vi "PyLoN_SRS5.vi"() -> ()   [LabVIEW 2014]
uses:
  Public/Documents/SIToolkit/LabVIEW/Examples2014_6_0_2_9/Fast Examples/Open-Close Hardware/CamHandle.vi
  <vilib>/Utility/file.llb/Write To Spreadsheet File (I64).vi
  <vilib>/Utility/file.llb/Write To Spreadsheet File (DBL).vi
panel:
  in  "Tab Control":enum32{"Page 1", "Page 2"}(tab)
  in  "Set camera":bool
  in  "stop":bool
  in  "Camera Number":u32=1
  in  "Write Tab Control":T1(tab)
  in  "Frames to collect (nframe)":u32=20000 min=1 step=1
  in  "Apply Timing":bool
  in  "Exposure":dbl min=0.0 step=0.001 format="%.3f"
  in  "Timing Mode":u32(ring)=1 items=["Free Run/Timed"=1, "External Sync/Strobed/Readout per Trigger"=3, "Shift per Trigger (kinetics only)"=13]
  in  "Trigger Edge":u32(ring)=1 items=["Positive Edge"=1, "Negative Edge"=2]
  in  "Collection Mode":u32(ring)=2 items=["Focus"=1, "N-Frame"=2, "Asynchronous"=3]
  in  "ReadOut Mode":u16(ring)=1 items=["Full Frame"=1, "Kinetics"=10]
  in  "Apply Temperature":bool
  in  "Temperature":dbl=-10.0 format="%.2f"
  in  "Apply ADC":bool
  in  "Speed":i32=-2 min=-3 step=1
  in  "Gain":i32(ring)=-1 items=["Don't Change "=-1, "Low"=1, "Medium"=2, "High"=3]
  in  "Offset":i32=-1 min=-1 step=1
  in  "Readout Port":i32(ring)=2 items=["Don't Change"=-1, "Low Noise"=1, "High capacity"=2]
  in  "Apply Shutter":bool
  in  "Open":u32
  in  "Close":u32
  in  "Shutter State":u16(ring)=3 items=["Always Closed"=1, "Open Each Exposure"=2, "Open at Begining of Acquisition"=3, "Open While Waiting for Trigger"=4]
  in  "Apply Cleans":bool
  in  "Final Section Height\n(Minimum Block Size)":u32=100
  in  "Final Section Count\n(Number of Minimum Blocks)":u32=10
  in  "Number of Clean/Clears cycles":u32
  in  "Clean cycle height (Number of \nStrips per Clean/Clear)":u32=100
  in  "Continous Cleans":bool
  in  "Skip Serial Register Clean":bool
  in  "Kinetics Window Height":u32
  in  "Active Y Size":u32=20
  in  "Post Y":u32
  in  "Pre Y":u32
  in  "Active X Size":u32=1340
  in  "Post X":u32
  in  "Pre X":u32
  in  "Vertical Timing Index":u32=1
  in  "Enable / Disable Custom Chip":bool=TRUE
  in  "Apply Custom Chip":bool
  in  "Apply Logic Out":bool
  in  "Logic Output":u16(ring)=1 items=["Not Scan / Not Reading"=1, "Shutter Open"=2, "Not Ready/Busy"=3, "Always Low"=4, "Always High"=8]
  in  "Invert":bool
  in  "Apply ROI":bool
  out "Y Size ROI":u32=20
  out "X Size ROI":u32=1340
  in  "Y Bin":u32=20 min=1 step=1
  in  "Y End":u32=20 min=1 step=1
  in  "Y Start":u32=1 min=1 step=1
  in  "X Bin":u32=1 min=1 step=1
  in  "X End":u32=1340 min=1 max=100000 step=1
  in  "X Start":u32=1 min=1 step=1
  in  "Write Status":string="Ready"
  out "Readout Time":dbl=0.8070999999999999
  in  "Read Camera settings":bool
  out "Temperature 2":dbl=-15.0
  out "Pixel Time\n(1/ADC Speed)":i32=500
  out "Bit Depth":i32=16
  out "ReadOut Port":i32=-1
  out "ADC Offset":i32=-1
  out "ADC Gain":i32=2
  out "ADC Speed":i32=2000
  out "Thermometer":dbl(slide)=-15.0 scale=-100.0..25.0 scale format="%#_6f"
  in  "Read Status":string="Ready"
  out "Camera Ready":bool=TRUE
  out "Vertical Timing":dbl=6.2
  out "Custom Chip Enabled":bool=TRUE
  out "Vertical Index":u32=1
  out "Frame Rate Calc":dbl=1239.003840911907
  in  "Clear Errors":bool
  in  "?":T2(tab)
  in  "?":bool
  in  "Exposure Time (s)":dbl=0.004 min=0.0 step=0.001 format="%.3f"
  in  "?":bool
  in  "?":bool
  out "?":u16[](graph)
  in  "file path":path
  in  "File_name":string
  in  "# of spectrum per frame":i32
  in  "# of Frames":i32
  in  "FLIP SPECTRA":bool
  in  "?":bool
  in  "?":bool
  in  "?":bool
  out "?":dbl[](graph)
  in  "?":bool
  in  "Number of Images":u32=1 min=1 step=1
  out "?":dbl[](graph)
  in  "?":bool
  in  "# of Sets":i32
  out "Current Set":u32=24
  in  "#Ground per set":u32=3
  in  "Timepoints":dbl[](array[numeric])=[200.0, 100.0, 300.0, 400.0, 500.0]
  in  "File Path":path
  in  "File Name":string
  in  "Ground State\nSubstract?":bool
  out "PyLoN Error Out":errorcluster
  out "PyLoN Ready":bool
  out "x/y":dbl
  in  "?":bool
  in  "Write INI Flag":bool
  out "error out":errorcluster
  in  "error in (no error)":errorcluster
  # "Write To Camera"
  # "Read From Camera"
  # "-1 = Item is not supported by this camera"
  # "ms"
  # "°C"
  # "ms"
  # "Timing"
  # "Seconds"
  # "Temperature"
  # "°C"
  # "ADC"
  # "-3 = SLOWEST speed\n-2 = FASTEST speed\n-1 = CURRENT speed (or do not wire)\nOtherwise enter speed in kHz"
  # "Shutter"
  # "Compensation Times"
  # "ms"
  # "Cleans / Clears"
  # "Custom Chip and Timing"
  # "Valid When Kinetics Timing Mode Active"
  # "Logic Output"
  # "Region Of Interest"
  # "REGION OF INTEREST"
  # "TRIGGER"
  # "ADC"
  # "SHUTTER"
  # "INPUT VARIABLES"
  # "TTL LOGIC"
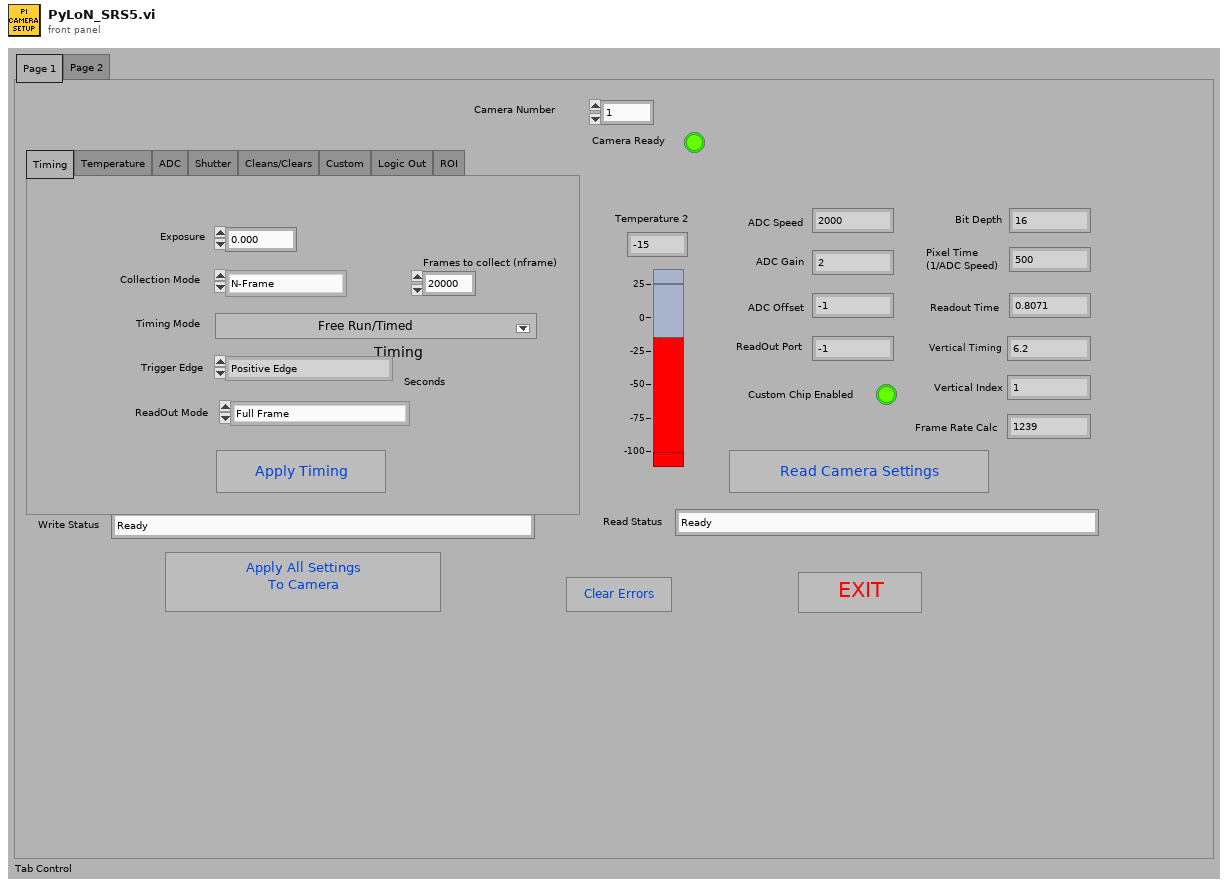
[diagram p1: front panel]
types:
  T1 = enum32{"Timing", "Temperature", "ADC", "Shutter", "Cleans/Clears", "Custom", "Logic Out", "ROI"}
  T2 = enum32{"CONFIGURATION", "RUN", "FOCUS", "FSRS", "SPECTROGRAPH", "ERROR"}
  T3 = cluster{"Pre Y":u32, "Post Y":u32, "Parallel (Y) Size":u32, "Pre X":u32, "Post X":u32, "Serial (X) Size":u32}
  T4 = cluster{"Camera Number":i32, "ROI Number":i32, "X Start":i32, "X End":i32, "X Bin":i32, "Y Start":i32, "Y End":i32, "Y Bin":i32}
  T5 = cluster{"Pre Y":u32, "Post Y":u32, "Active Y":u32, "Pre X":u32, "Post X":u32, "Active X":u32, "Custom Chip Enabled":bool, "Vertical Timing Index":u32}
  T6 = cluster{"Exposure":dbl, "Collection Mode":u32, "Timing Mode":u32, "Trigger Edge":u32, "Temperature":dbl}
  T7 = cluster{"ADC Speed":i32, "ADC Gain":i32, "ADC Offset":i32, "Readout Port":i32, "Num Cleans":u32, "Num Strips per Clean":u32, "Mini Block Size":u32, "Num Min Blocks":u32, "Continous Cleans":bool, "Skip Serial Reg Clean":bool}
  T8 = cluster{"Shutter State":u16, "Open Comp Time ":u32, "Close Comp Time":u32, "Logic Out Setting":u32, "Logic Out Invert":bool}
  T9 = enum32{"Initializing", "RUN", "FSRS", "Monochromator", "Errors"}
  T10 = cluster{"X Start":i32, "X End":i32, "X Bin":i32, "Y Start":i32, "Y End":i32, "Y Bin":i32}
  T11 = cluster{"Value":u32, "Value":u32, "Value":u32, "Value":u32, "Value":u32, "Value":u32}
  T12 = cluster{"acquire focus mode":u32, "Exposure Time (s)":dbl, i32, "Software accumulation":u32}
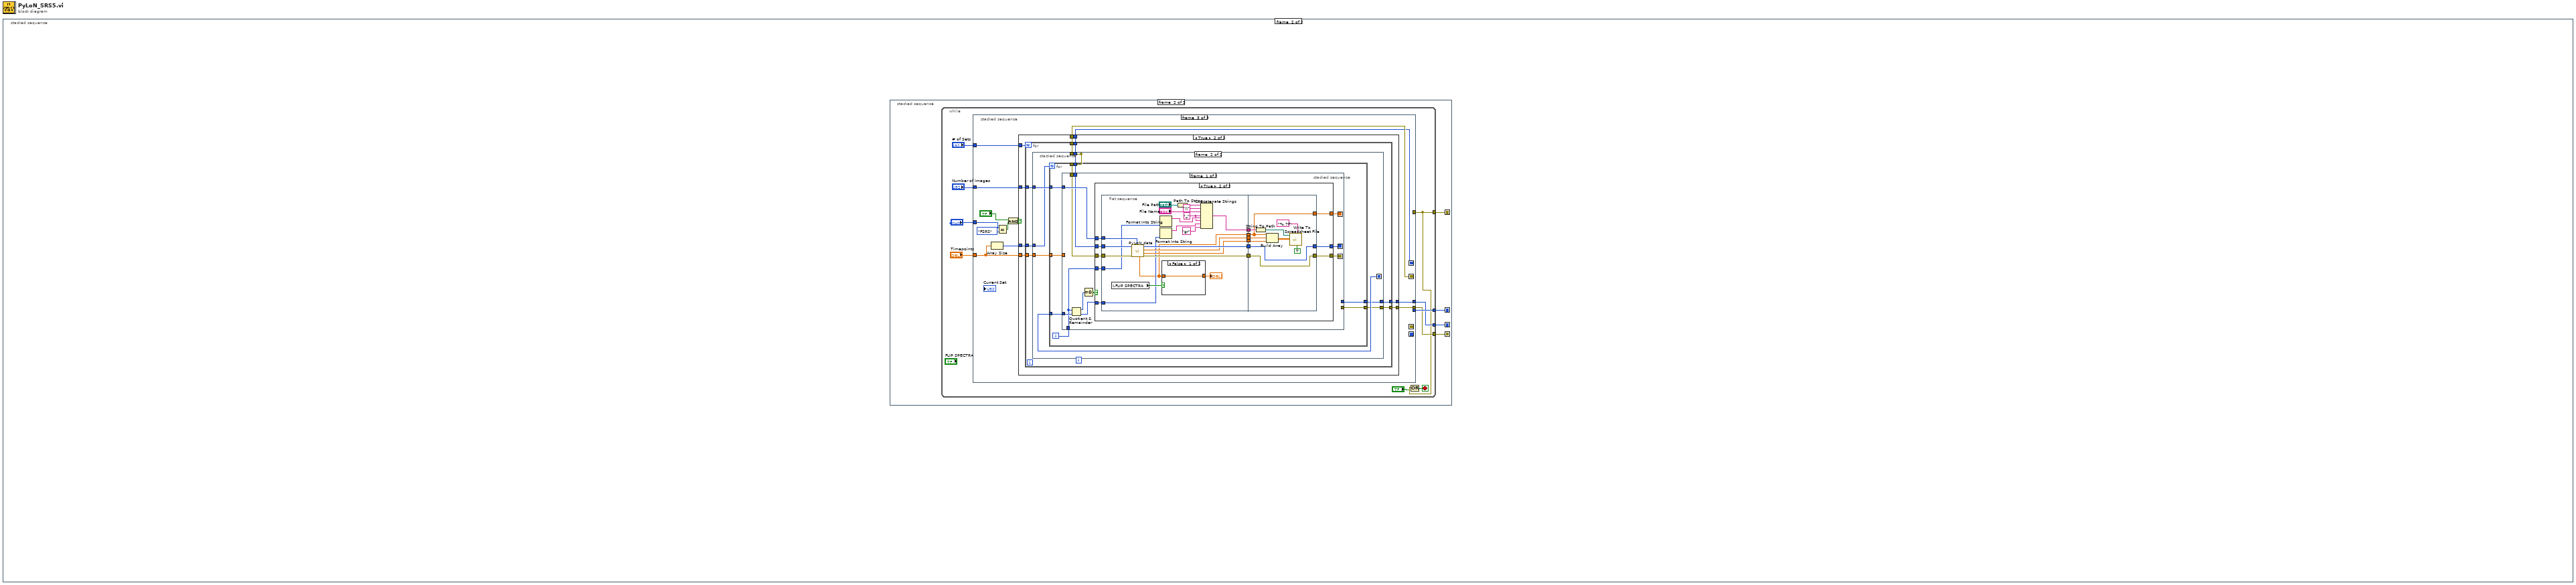
[diagram p0: block diagram]
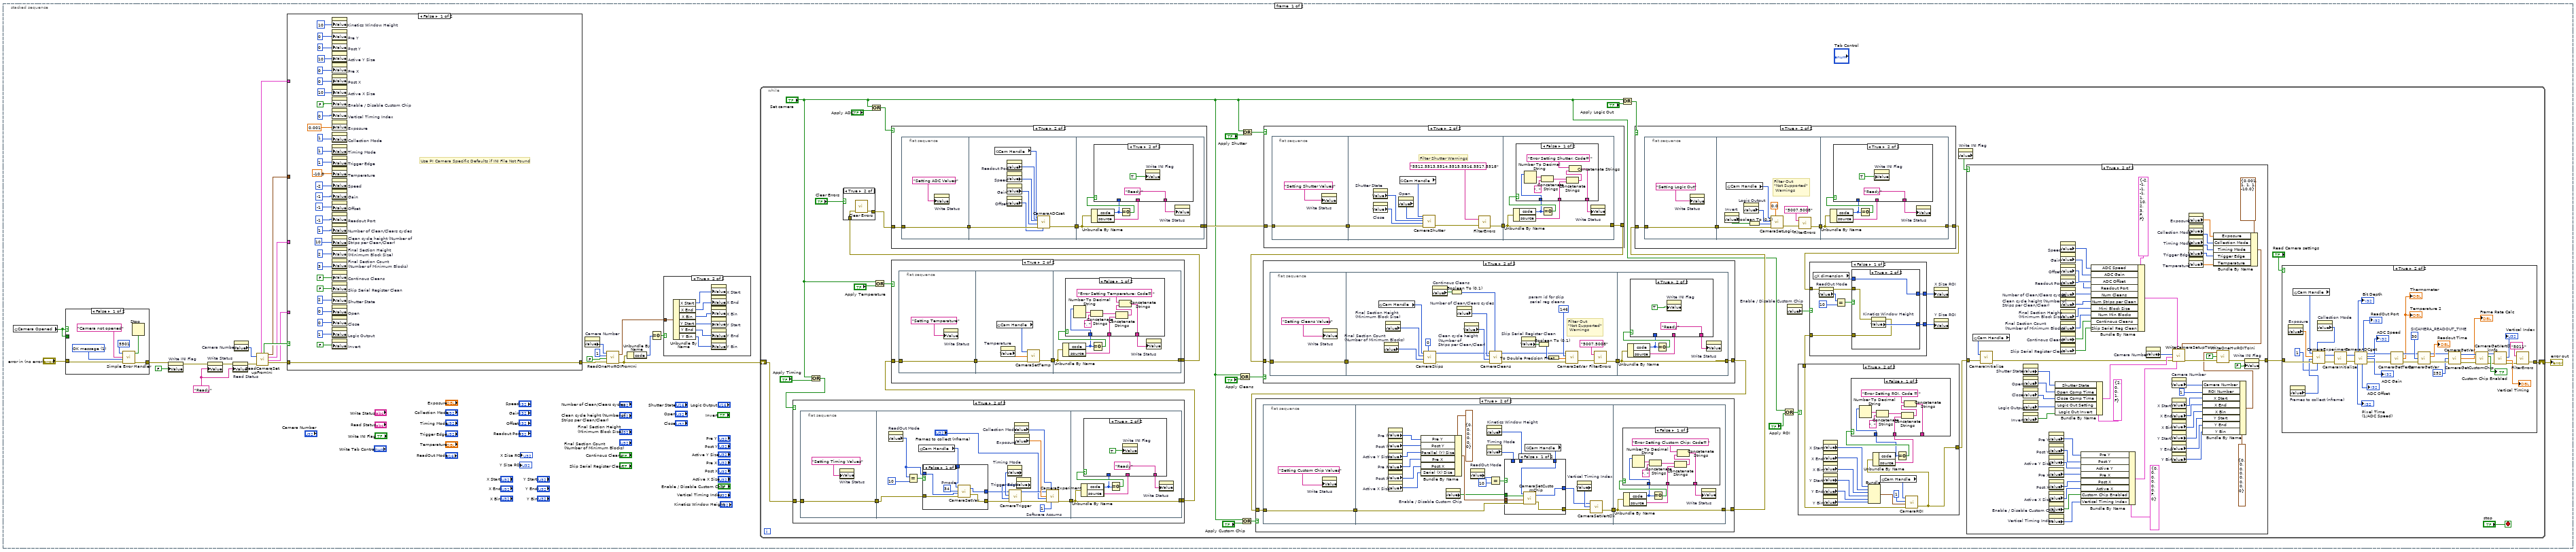
[diagram p2: hidden frame]
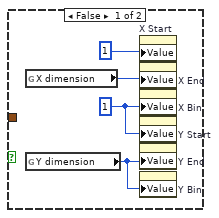
[diagram p3: hidden frame]
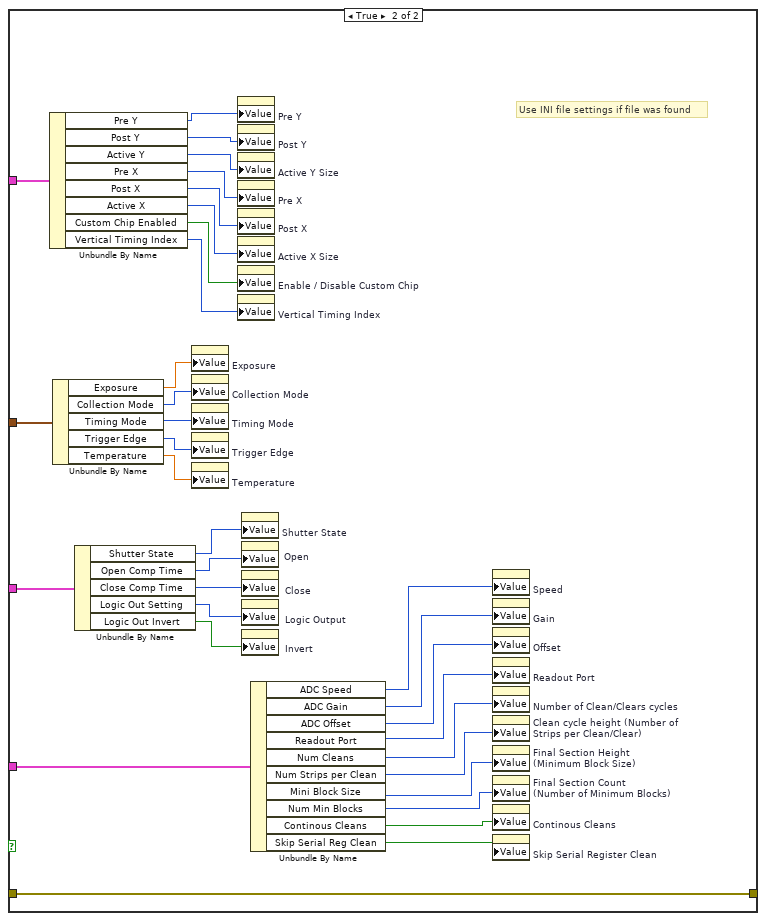
[diagram p4: hidden frame]
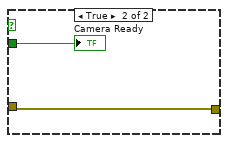
[diagram p5: hidden frame]
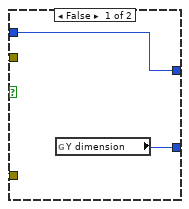
[diagram p7: hidden frame]
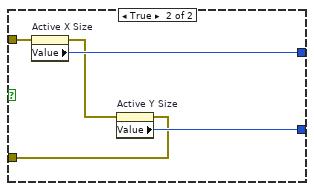
[diagram p8: hidden frame]
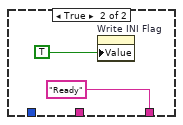
[diagram p10: hidden frame]
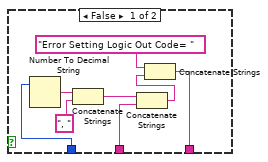
[diagram p12: hidden frame]
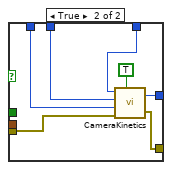
[diagram p14: hidden frame]
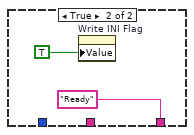
[diagram p15: hidden frame]
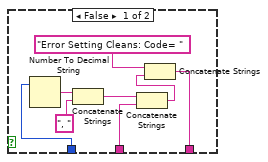
[diagram p17: hidden frame]
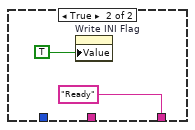
[diagram p19: hidden frame]
diagram:
  n1 = stacked-sequence {
    frame #0 {
      w15 = "Ready"
      n2 = global read "CamHandle.vi" "Camera Opened"() -> (w11:bool)
      n3 = case shown="False" w11 {
        tunnel: [w103 w106] -> w14
        tunnel: "error in (no error)" -> [w99 w106]
        tunnel: w11 -> [_ w105]
        frame False {
          w104 = u16 1 items=["no dialog", "OK message", "continue or stop message"] ("type of dialog (OK msg:1)")
          n4 = call <vilib>:"Simple Error Handler.vi"("error code (no error:0)"=5501, "error source (\" \")"="Camera not opened", "type of dialog (OK msg:1)"=w104, "error in (no error)"=w99) -> ("error?"=w101:bool, "error out"=w103:errorcluster)  [unwired: 1 in, 3 out]
          n5 = Stop(stop? (T)=w101) -> ()
        }
        frame True {
          "Camera Ready" <- w105
        }
      }
      n6 = property on="Write INI Flag" class="Bool (strict)"(error in=w14, "Value"=FALSE) -> (error out=w13:errorcluster)  [unwired: 1 in, 1 out]
      n7 = property on="Write Status" class="Str"(error in=w13, "Value"=w15) -> (error out=w17:errorcluster)  [unwired: 1 in, 1 out]
      n8 = property on="Read Status" class="Str"(error in=w17, "Value"=w15) -> (error out=w16:errorcluster)  [unwired: 1 in, 1 out]
      n9 = property on="Camera Number" class="DigNum (strict)"() -> ("Value"=w8:u32)  [unwired: 2 in, 2 out]
      n10 = call "ReadCameraSetupFromIni.vi"("error in (no error)"=w16, "Camera Number"=w8) -> ("Custom Chip"=w10:T5, "INI File Found"=w22:bool, "error out"=w18:errorcluster, "ADC and Cleans"=w21:T7, "Shutter and Logic Out"=w20:T8, "Timing and Temperature"=w19:T6)
      n11 = case shown="False" w22 {
        tunnel: w19 -> [_ w98]
        tunnel: w20 -> [_ w92]
        tunnel: w21 -> [_ w86]
        tunnel: w18 -> [w45 w75]
        tunnel: [w45 w75] -> w9
        tunnel: w10 -> [_ w74]
        frame False {
          # "Use PI Camera Specific Defaults if INI File Not Found"
          n12 = property on="Kinetics Window Height" class="DigNum (strict)"("Value"=10) -> ()  [unwired: 2 in, 2 out]
          n13 = property on="Pre Y" class="DigNum (strict)"("Value"=0) -> ()  [unwired: 2 in, 2 out]
          n14 = property on="Post Y" class="DigNum (strict)"("Value"=0) -> ()  [unwired: 2 in, 2 out]
          n15 = property on="Active Y Size" class="DigNum (strict)"("Value"=10) -> ()  [unwired: 2 in, 2 out]
          n16 = property on="Pre X" class="DigNum (strict)"("Value"=0) -> ()  [unwired: 2 in, 2 out]
          n17 = property on="Post X" class="DigNum (strict)"("Value"=0) -> ()  [unwired: 2 in, 2 out]
          n18 = property on="Active X Size" class="DigNum (strict)"("Value"=10) -> ()  [unwired: 2 in, 2 out]
          n19 = property on="Enable / Disable Custom Chip" class="Bool (strict)"("Value"=FALSE) -> ()  [unwired: 2 in, 2 out]
          n20 = property on="Vertical Timing Index" class="DigNum (strict)"("Value"=0) -> ()  [unwired: 2 in, 2 out]
          n21 = property on="Exposure" class="DigNum (strict)"("Value"=0.001 ("Exposure")) -> ()  [unwired: 2 in, 2 out]
          n22 = property on="Collection Mode" class="Ring (strict)"("Value"=u32 1 ("Collection Mode")) -> ()  [unwired: 2 in, 2 out]
          n23 = property on="Timing Mode" class="Ring (strict)"("Value"=u32 1 ("Timing Mode")) -> ()  [unwired: 2 in, 2 out]
          n24 = property on="Trigger Edge" class="Ring (strict)"("Value"=u32 1 ("Trigger Edge")) -> ()  [unwired: 2 in, 2 out]
          n25 = property on="Temperature" class="DigNum (strict)"("Value"=-10.0 ("Temperature")) -> ()  [unwired: 2 in, 2 out]
          n26 = property on="Speed" class="DigNum (strict)"("Value"=-2 ("ADC Speed")) -> ()  [unwired: 2 in, 2 out]
          n27 = property on="Gain" class="Ring (strict)"("Value"=-1 ("ADC Gain")) -> ()  [unwired: 2 in, 2 out]
          n28 = property on="Offset" class="DigNum (strict)"("Value"=-1 ("ADC Offset")) -> ()  [unwired: 2 in, 2 out]
          n29 = property on="Readout Port" class="Ring (strict)"("Value"=-1 ("Readout Port")) -> ()  [unwired: 2 in, 2 out]
          n30 = property on="Number of Clean/Clears cycles" class="DigNum (strict)"("Value"=u32 1 ("Num Cleans")) -> ()  [unwired: 2 in, 2 out]
          n31 = property on="Clean cycle height (Number of \nStrips per Clean/Clear)" class="DigNum (strict)"("Value"=u32 10 ("Num Strips per Clean")) -> ()  [unwired: 2 in, 2 out]
          n32 = property on="Final Section Height\n(Minimum Block Size)" class="DigNum (strict)"("Value"=u32 2 ("Mini Block Size")) -> ()  [unwired: 2 in, 2 out]
          n33 = property on="Final Section Count\n(Number of Minimum Blocks)" class="DigNum (strict)"("Value"=u32 3 ("Num Min Blocks")) -> ()  [unwired: 2 in, 2 out]
          n34 = property on="Continous Cleans" class="Bool (strict)"("Value"=FALSE ("Continous Cleans")) -> ()  [unwired: 2 in, 2 out]
          n35 = property on="Skip Serial Register Clean" class="Bool (strict)"("Value"=FALSE ("Skip Serial Reg Clean")) -> ()  [unwired: 2 in, 2 out]
          n36 = property on="Shutter State" class="Ring (strict)"("Value"=u16 2 ("Shutter State")) -> ()  [unwired: 2 in, 2 out]
          n37 = property on="Open" class="DigNum (strict)"("Value"=u32 0 ("Open Comp Time")) -> ()  [unwired: 2 in, 2 out]
          n38 = property on="Close" class="DigNum (strict)"("Value"=u32 0 ("Close Comp Time")) -> ()  [unwired: 2 in, 2 out]
          n39 = property on="Logic Output" class="Ring (strict)"("Value"=u32 1 ("Logic Out Setting")) -> ()  [unwired: 2 in, 2 out]
          n40 = property on="Invert" class="Bool (strict)"("Value"=FALSE ("Logic Out Invert")) -> ()  [unwired: 2 in, 2 out]
        }
        frame True {
          # "Use INI file settings if file was found"
          n41 = Unbundle By Name(w74) -> ("Pre Y"=w73:u32, "Post Y"=w71:u32, "Active Y"=w70:u32, "Pre X"=w69:u32, "Post X"=w72:u32, "Active X"=w68:u32, "Custom Chip Enabled"=w67:bool, "Vertical Timing Index"=w66:u32)
          n42 = Unbundle By Name(w98) -> ("Exposure"=w97:dbl, "Collection Mode"=w96:u32, "Timing Mode"=w95:u32, "Trigger Edge"=w94:u32, "Temperature"=w93:dbl)
          n43 = Unbundle By Name(w92) -> ("Shutter State"=w91:u16, "Open Comp Time"=w90:u32, "Close Comp Time"=w89:u32, "Logic Out Setting"=w88:u32, "Logic Out Invert"=w87:bool)
          n44 = property on="Exposure" class="DigNum (strict)"("Value"=w97) -> ()  [unwired: 2 in, 2 out]
          n45 = property on="Collection Mode" class="Ring (strict)"("Value"=w96) -> ()  [unwired: 2 in, 2 out]
          n46 = property on="Timing Mode" class="Ring (strict)"("Value"=w95) -> ()  [unwired: 2 in, 2 out]
          n47 = property on="Trigger Edge" class="Ring (strict)"("Value"=w94) -> ()  [unwired: 2 in, 2 out]
          n48 = property on="Temperature" class="DigNum (strict)"("Value"=w93) -> ()  [unwired: 2 in, 2 out]
          n49 = property on="Pre Y" class="DigNum (strict)"("Value"=w73) -> ()  [unwired: 2 in, 2 out]
          n50 = property on="Post Y" class="DigNum (strict)"("Value"=w71) -> ()  [unwired: 2 in, 2 out]
          n51 = property on="Active Y Size" class="DigNum (strict)"("Value"=w70) -> ()  [unwired: 2 in, 2 out]
          n52 = property on="Pre X" class="DigNum (strict)"("Value"=w69) -> ()  [unwired: 2 in, 2 out]
          n53 = property on="Post X" class="DigNum (strict)"("Value"=w72) -> ()  [unwired: 2 in, 2 out]
          n54 = property on="Active X Size" class="DigNum (strict)"("Value"=w68) -> ()  [unwired: 2 in, 2 out]
          n55 = property on="Enable / Disable Custom Chip" class="Bool (strict)"("Value"=w67) -> ()  [unwired: 2 in, 2 out]
          n56 = property on="Vertical Timing Index" class="DigNum (strict)"("Value"=w66) -> ()  [unwired: 2 in, 2 out]
          n57 = property on="Shutter State" class="Ring (strict)"("Value"=w91) -> ()  [unwired: 2 in, 2 out]
          n58 = property on="Open" class="DigNum (strict)"("Value"=w90) -> ()  [unwired: 2 in, 2 out]
          n59 = property on="Close" class="DigNum (strict)"("Value"=w89) -> ()  [unwired: 2 in, 2 out]
          n60 = property on="Logic Output" class="Ring (strict)"("Value"=w88) -> ()  [unwired: 2 in, 2 out]
          n61 = property on="Invert" class="Bool (strict)"("Value"=w87) -> ()  [unwired: 2 in, 2 out]
          n62 = Unbundle By Name(w86) -> ("ADC Speed"=w76:i32, "ADC Gain"=w77:i32, "ADC Offset"=w78:i32, "Readout Port"=w79:i32, "Num Cleans"=w80:u32, "Num Strips per Clean"=w81:u32, "Mini Block Size"=w82:u32, "Num Min Blocks"=w83:u32, "Continous Cleans"=w84:bool, "Skip Serial Reg Clean"=w85:bool)
          n63 = property on="Speed" class="DigNum (strict)"("Value"=w76) -> ()  [unwired: 2 in, 2 out]
          n64 = property on="Gain" class="Ring (strict)"("Value"=w77) -> ()  [unwired: 2 in, 2 out]
          n65 = property on="Offset" class="DigNum (strict)"("Value"=w78) -> ()  [unwired: 2 in, 2 out]
          n66 = property on="Readout Port" class="Ring (strict)"("Value"=w79) -> ()  [unwired: 2 in, 2 out]
          n67 = property on="Number of Clean/Clears cycles" class="DigNum (strict)"("Value"=w80) -> ()  [unwired: 2 in, 2 out]
          n68 = property on="Clean cycle height (Number of \nStrips per Clean/Clear)" class="DigNum (strict)"("Value"=w81) -> ()  [unwired: 2 in, 2 out]
          n69 = property on="Final Section Height\n(Minimum Block Size)" class="DigNum (strict)"("Value"=w82) -> ()  [unwired: 2 in, 2 out]
          n70 = property on="Final Section Count\n(Number of Minimum Blocks)" class="DigNum (strict)"("Value"=w83) -> ()  [unwired: 2 in, 2 out]
          n71 = property on="Continous Cleans" class="Bool (strict)"("Value"=w84) -> ()  [unwired: 2 in, 2 out]
          n72 = property on="Skip Serial Register Clean" class="Bool (strict)"("Value"=w85) -> ()  [unwired: 2 in, 2 out]
        }
      }
      n73 = property on="Camera Number" class="DigNum (strict)"() -> ("Value"=w7:u32)  [unwired: 2 in, 2 out]
      n74 = call "ReadOneHwROIFromIni.vi"("error in (no error)"=w9, "Show Message"=FALSE, "ROI Number"=1, "Camera Number"=w7) -> ("error out"=w4:errorcluster, "ROI Values"=w1:T10)
      n75 = Unbundle By Name(w4) -> ("code"=w2:i32)
      n76 = Equal To 0?(x=w2) -> (x = 0?=w3:bool)
      n77 = case shown="True" w3 {
        tunnel: w1 -> [_ w35]
        frame False {
          w26 = 1
          n78 = global read "CamHandle.vi" "X dimension"() -> (w27:u32)
          n79 = global read "CamHandle.vi" "Y dimension"() -> (w25:u32)
          n80 = property on="X Start" class="DigNum (strict)"("Value"=1) -> ()  [unwired: 2 in, 2 out]
          n81 = property on="X End" class="DigNum (strict)"("Value"=w27) -> ()  [unwired: 2 in, 2 out]
          n82 = property on="X Bin" class="DigNum (strict)"("Value"=w26) -> ()  [unwired: 2 in, 2 out]
          n83 = property on="Y Start" class="DigNum (strict)"("Value"=w26) -> ()  [unwired: 2 in, 2 out]
          n84 = property on="Y End" class="DigNum (strict)"("Value"=w25) -> ()  [unwired: 2 in, 2 out]
          n85 = property on="Y Bin" class="DigNum (strict)"("Value"=w25) -> ()  [unwired: 2 in, 2 out]
        }
        frame True {
          n86 = Unbundle By Name(w35) -> ("X Start"=w34:i32, "X End"=w33:i32, "X Bin"=w32:i32, "Y Start"=w31:i32, "Y End"=w30:i32, "Y Bin"=w29:i32)
          n87 = property on="X Start" class="DigNum (strict)"("Value"=w34) -> ()  [unwired: 2 in, 2 out]
          n88 = property on="X End" class="DigNum (strict)"("Value"=w33) -> ()  [unwired: 2 in, 2 out]
          n89 = property on="X Bin" class="DigNum (strict)"("Value"=w32) -> ()  [unwired: 2 in, 2 out]
          n90 = property on="Y Start" class="DigNum (strict)"("Value"=w31) -> ()  [unwired: 2 in, 2 out]
          n91 = property on="Y End" class="DigNum (strict)"("Value"=w30) -> ()  [unwired: 2 in, 2 out]
          n92 = property on="Y Bin" class="DigNum (strict)"("Value"=w29) -> ()  [unwired: 2 in, 2 out]
        }
      }
      n93 = while {
        shift-right: [w141] -> w23
        shift-left: w4 -> [w137]
        stop <- "stop" stop-if-true
        n94 = Or(x="Set camera", y="Apply Timing") -> (x .or. y?=w138:bool)
        n95 = case shown="True" w138 {
          tunnel: w137 -> [w463 w467]
          tunnel: [w463 w464] -> w135
          frame False {
          }
          frame True {
            n96 = flat-sequence {
              tunnel: w467 -> [w469]
              tunnel: [w469] -> w466
              tunnel: w466 -> [w474]
              tunnel: [w478] -> w465
              tunnel: w465 -> [w498]
              tunnel: [w498] -> w464
              frame #0 {
                n97 = property on="Write Status" class="Str"("Value"="Setting Timing Values") -> ()  [unwired: 2 in, 2 out]
              }
              frame #1 {
                w483 = 1  # Software Accums
                n98 = property on="ReadOut Mode" class="Ring (strict)"() -> ("Value"=w471:u16)  [unwired: 2 in, 2 out]
                n99 = Equal?(x=w471, y=10) -> (x = y?=w473:bool)
                n100 = global read "CamHandle.vi" "Cam Handle"() -> (w475:u32)
                n101 = case shown="False" w473 {
                  tunnel: [w490 w492] -> w477
                  tunnel: [w489 w493] -> w476
                  tunnel: w475 -> [w488 w493]
                  tunnel: w474 -> [w487 w492]
                  tunnel: w471 -> [w486 _]
                  frame False {
                    w491 = 34  # Pmode
                    n102 = call <userlib>:"CameraSetVar.vi"("error in"=w487, "Value"=w486, "Parameter ID"=w491, "Camera Handle"=w488) -> ("error out"=w490:errorcluster, "CameraHandle"=w489:u32)
                  }
                  frame True {
                  }
                }
                n103 = property on="Timing Mode" class="Ring (strict)"() -> ("Value"=w485:u32)  [unwired: 2 in, 2 out]
                n104 = property on="Collection Mode" class="Ring (strict)"() -> ("Value"=w482:u32)  [unwired: 2 in, 2 out]
                n105 = property on="Exposure" class="DigNum (strict)"() -> ("Value"=w484:dbl)  [unwired: 2 in, 2 out]
                n106 = property on="Trigger Edge" class="Ring (strict)"() -> ("Value"=w480:u32)  [unwired: 2 in, 2 out]
                n107 = call <userlib>:"CameraTrigger.vi"("error in"=w477, "Trigger Edge"=w480, "Timing Mode"=w485, "Camera Handle"=w476) -> ("error out"=w479:errorcluster, "Camera Handle"=w481:u32)
                n108 = call <userlib>:"CameraExperiment.vi"("Number of Accumulations"=w483, "Acquire / Focus Flag"=w482, "error in"=w479, "Number of Images"="Frames to collect (nframe)", "Exposure (sec)"=w484, "Camera Handle"=w481) -> ("error out"=w478:errorcluster)  [unwired: 1 out]
              }
              frame #2 {
                n109 = Unbundle By Name(w498) -> ("code"=w494:i32, "source"=w495:string)
                n110 = Equal To 0?(x=w494) -> (x = 0?=w497:bool)
                n111 = case shown="True" w497 {
                  tunnel: [w499 "Ready"] -> w496
                  tunnel: w495 -> [w500 _]
                  tunnel: w494 -> [w505 _]
                  frame False {
                    n112 = Number To Decimal String(number=w505) -> (decimal integer string=w504:string)  [unwired: 1 in]
                    n113 = Concatenate Strings(w504, ", ") -> (w501:string)
                    n114 = Concatenate Strings(w501, w500) -> (w502:string)
                    n115 = Concatenate Strings("Error Setting Timing: Code= ", w502) -> (w499:string)
                  }
                  frame True {
                    n116 = property on="Write INI Flag" class="Bool (strict)"("Value"=TRUE) -> ()  [unwired: 2 in, 2 out]
                  }
                }
                n117 = property on="Write Status" class="Str"("Value"=w496) -> ()  [unwired: 2 in, 2 out]
              }
            }
          }
        }
        n118 = Or(x="Set camera", y="Apply ADC") -> (x .or. y?=w133:bool)
        n119 = Or(x="Set camera", y="Apply Temperature") -> (x .or. y?=w136:bool)
        n120 = case shown="True" w136 {
          tunnel: w135 -> [w437 w441]
          tunnel: [w437 w438] -> w111
          frame False {
          }
          frame True {
            n121 = flat-sequence {
              tunnel: w441 -> [w443]
              tunnel: [w443] -> w440
              tunnel: w440 -> [w445]
              tunnel: [w444] -> w439
              tunnel: w439 -> [w452]
              tunnel: [w452] -> w438
              frame #0 {
                n122 = property on="Write Status" class="Str"("Value"="Setting Temperature") -> ()  [unwired: 2 in, 2 out]
              }
              frame #1 {
                n123 = global read "CamHandle.vi" "Cam Handle"() -> (w446:u32)
                n124 = property on="Temperature" class="DigNum (strict)"() -> ("Value"=w447:dbl)  [unwired: 2 in, 2 out]
                n125 = call <userlib>:"CameraSetTemp.vi"("error in (no error)"=w445, "Temperature"=w447, "Camera Handle"=w446) -> ("error out"=w444:errorcluster)  [unwired: 1 out]
              }
              frame #2 {
                n126 = Unbundle By Name(w452) -> ("code"=w449:i32, "source"=w450:string)
                n127 = Equal To 0?(x=w449) -> (x = 0?=w451:bool)
                n128 = case shown="False" w451 {
                  tunnel: [w453 "Ready"] -> w448
                  tunnel: w450 -> [w454 _]
                  tunnel: w449 -> [w459 _]
                  frame False {
                    n129 = Number To Decimal String(number=w459) -> (decimal integer string=w458:string)  [unwired: 1 in]
                    n130 = Concatenate Strings(w458, ", ") -> (w455:string)
                    n131 = Concatenate Strings(w455, w454) -> (w456:string)
                    n132 = Concatenate Strings("Error Setting Temperature: Code= ", w456) -> (w453:string)
                  }
                  frame True {
                    n133 = property on="Write INI Flag" class="Bool (strict)"("Value"=TRUE) -> ()  [unwired: 2 in, 2 out]
                  }
                }
                n134 = property on="Write Status" class="Str"("Value"=w448) -> ()  [unwired: 2 in, 2 out]
              }
            }
          }
        }
        n135 = case shown="True" "Clear Errors" {
          tunnel: w111 -> [w144 w146]
          tunnel: [w144 w145] -> w110
          frame False {
          }
          frame True {
            n136 = call <vilib>:"Clear Errors.vi"("error in (no error)"=w146) -> ("error out"=w145:errorcluster)  [unwired: 5 in, 1 out]
          }
        }
        n137 = case shown="True" w133 {
          tunnel: w110 -> [w351 w355]
          tunnel: [w351 w352] -> w132
          frame False {
          }
          frame True {
            n138 = flat-sequence {
              tunnel: w355 -> [w357]
              tunnel: [w357] -> w354
              tunnel: w354 -> [w361]
              tunnel: [w360] -> w353
              tunnel: w353 -> [w366]
              tunnel: [w366] -> w352
              frame #0 {
                n139 = property on="Write Status" class="Str"("Value"="Setting ADC Values") -> ()  [unwired: 2 in, 2 out]
              }
              frame #1 {
                n140 = global read "CamHandle.vi" "Cam Handle"() -> (w358:u32)
                n141 = property on="Readout Port" class="Ring (strict)"() -> ("Value"=w362:i32)  [unwired: 2 in, 2 out]
                n142 = property on="Speed" class="DigNum (strict)"() -> ("Value"=w363:i32)  [unwired: 2 in, 2 out]
                n143 = property on="Gain" class="Ring (strict)"() -> ("Value"=w364:i32)  [unwired: 2 in, 2 out]
                n144 = property on="Offset" class="DigNum (strict)"() -> ("Value"=w359:i32)  [unwired: 2 in, 2 out]
                n145 = call <userlib>:"CameraADCset.vi"("ADC offset"=w359, "Read Out port"=w362, "error in (no error)"=w361, "ADC Gain"=w364, "ADC Speed"=w363, "Camera Handle"=w358) -> ("error out"=w360:errorcluster)  [unwired: 1 out]
              }
              frame #2 {
                n146 = Unbundle By Name(w366) -> ("code"=w367:i32, "source"=w368:string)
                n147 = Equal To 0?(x=w367) -> (x = 0?=w369:bool)
                n148 = case shown="True" w369 {
                  tunnel: [w370 "Ready"] -> w365
                  tunnel: w368 -> [w371 _]
                  tunnel: w367 -> [w376 _]
                  frame False {
                    n149 = Number To Decimal String(number=w376) -> (decimal integer string=w375:string)  [unwired: 1 in]
                    n150 = Concatenate Strings(w375, ", ") -> (w372:string)
                    n151 = Concatenate Strings(w372, w371) -> (w373:string)
                    n152 = Concatenate Strings("Error Setting ADC: Code= ", w373) -> (w370:string)
                  }
                  frame True {
                    n153 = property on="Write INI Flag" class="Bool (strict)"("Value"=TRUE) -> ()  [unwired: 2 in, 2 out]
                  }
                }
                n154 = property on="Write Status" class="Str"("Value"=w365) -> ()  [unwired: 2 in, 2 out]
              }
            }
          }
        }
        n155 = Or(x="Set camera", y="Apply Cleans") -> (x .or. y?=w127:bool)
        n156 = Or(x="Set camera", y="Apply Custom Chip") -> (x .or. y?=w124:bool)
        n157 = Or(x="Set camera", y="Apply Shutter") -> (x .or. y?=w129:bool)
        n158 = case shown="True" w129 {
          tunnel: w132 -> [w321 w325]
          tunnel: [w321 w322] -> w128
          frame False {
          }
          frame True {
            n159 = flat-sequence {
              tunnel: w325 -> [w327]
              tunnel: [w327] -> w324
              tunnel: w324 -> [w331]
              tunnel: [w329] -> w323
              tunnel: w323 -> [w340]
              tunnel: [w340] -> w322
              frame #0 {
                n160 = property on="Write Status" class="Str"("Value"="Setting Shutter Values") -> ()  [unwired: 2 in, 2 out]
              }
              frame #1 {
                # "Filter Shutter Warnings"
                n161 = property on="Shutter State" class="Ring (strict)"() -> ("Value"=w334:u16)  [unwired: 2 in, 2 out]
                n162 = property on="Close" class="DigNum (strict)"() -> ("Value"=w332:u32)  [unwired: 2 in, 2 out]
                n163 = property on="Open" class="DigNum (strict)"() -> ("Value"=w333:u32)  [unwired: 2 in, 2 out]
                n164 = global read "CamHandle.vi" "Cam Handle"() -> (w328:u32)
                n165 = call <userlib>:"CameraShutter.vi"("Camera Handle"=w328, "Shutter Comp Time: Pre Open"=w333, "Shutter Comp Time: Post Open"=w332, "error in"=w331, "Shutter State"=w334) -> ("error out"=w330:errorcluster)  [unwired: 1 out]
                n166 = call "FilterErrors.vi"("error in (no error)"=w330, "Error Numbers To Filter"="5512,5513,5514,5515,5516,5517,5518") -> ("error out"=w329:errorcluster)
              }
              frame #2 {
                n167 = Unbundle By Name(w340) -> ("code"=w337:i32, "source"=w338:string)
                n168 = Equal To 0?(x=w337) -> (x = 0?=w339:bool)
                n169 = case shown="False" w339 {
                  tunnel: [w341 "Ready"] -> w336
                  tunnel: w338 -> [w342 _]
                  tunnel: w337 -> [w347 _]
                  frame False {
                    n170 = Number To Decimal String(number=w347) -> (decimal integer string=w346:string)  [unwired: 1 in]
                    n171 = Concatenate Strings(w346, ", ") -> (w343:string)
                    n172 = Concatenate Strings(w343, w342) -> (w344:string)
                    n173 = Concatenate Strings("Error Setting Shutter: Code= ", w344) -> (w341:string)
                  }
                  frame True {
                    n174 = property on="Write INI Flag" class="Bool (strict)"("Value"=TRUE) -> ()  [unwired: 2 in, 2 out]
                  }
                }
                n175 = property on="Write Status" class="Str"("Value"=w336) -> ()  [unwired: 2 in, 2 out]
              }
            }
          }
        }
        n176 = case shown="True" w127 {
          tunnel: w128 -> [w279 w283]
          tunnel: [w279 w280] -> w125
          frame False {
          }
          frame True {
            n177 = flat-sequence {
              tunnel: w283 -> [w285]
              tunnel: [w285] -> w282
              tunnel: w282 -> [w298]
              tunnel: [w286] -> w281
              tunnel: w281 -> [w310]
              tunnel: [w310] -> w280
              frame #0 {
                n178 = property on="Write Status" class="Str"("Value"="Setting Cleans Values") -> ()  [unwired: 2 in, 2 out]
              }
              frame #1 {
                w290 = u32 146  # param id for skip  serial reg cleans
                # "Filter Out\n\"Not Supported\"\n Warnings"
                n179 = global read "CamHandle.vi" "Cam Handle"() -> (w299:u32)
                n180 = property on="Final Section Count\n(Number of Minimum Blocks)" class="DigNum (strict)"() -> ("Value"=w304:u32)  [unwired: 2 in, 2 out]
                n181 = property on="Final Section Height\n(Minimum Block Size)" class="DigNum (strict)"() -> ("Value"=w305:u32)  [unwired: 2 in, 2 out]
                n182 = call <userlib>:"CameraSkips.vi"("Camera Handle"=w299, "Minimum Block Size"=w305, "Number of Minimum blocks"=w304, "error in"=w298, "Type of Skips"=u32 0) -> ("Camera Handle"=w295:u32, "error out"=w296:errorcluster)
                n183 = property on="Continous Cleans" class="Bool (strict)"() -> ("Value"=w302:bool)  [unwired: 2 in, 2 out]
                n184 = Boolean To (0,1)(Boolean=w302) -> (0, 1=w297:i16)
                n185 = property on="Number of Clean/Clears cycles" class="DigNum (strict)"() -> ("Value"=w301:u32)  [unwired: 2 in, 2 out]
                n186 = property on="Clean cycle height (Number of \nStrips per Clean/Clear)" class="DigNum (strict)"() -> ("Value"=w300:u32)  [unwired: 2 in, 2 out]
                n187 = call <userlib>:"CameraCleans.vi"("Camera Handle"=w295, "Number of Clears"=w301, "Number of Strips Per Clear"=w300, "error in"=w296, "Continuous Clears"=w297) -> ("Camera Handle"=w287:u32, "error out"=w288:errorcluster)
                n188 = property on="Skip Serial Register Clean" class="Bool (strict)"() -> ("Value"=w292:bool)  [unwired: 2 in, 2 out]
                n189 = Boolean To (0,1)(Boolean=w292) -> (0, 1=w291:i16)
                n190 = To Double Precision Float(number=w291) -> (double precision float=w293:dbl)
                n191 = call <userlib>:"CameraSetVar.vi"("error in"=w288, "Value"=w293, "Parameter ID"=w290, "Camera Handle"=w287) -> ("error out"=w289:errorcluster)  [unwired: 1 out]
                n192 = call "FilterErrors.vi"("error in (no error)"=w289, "Error Numbers To Filter"="5007,5008") -> ("error out"=w286:errorcluster)
              }
              frame #2 {
                n193 = Unbundle By Name(w310) -> ("code"=w307:i32, "source"=w308:string)
                n194 = Equal To 0?(x=w307) -> (x = 0?=w309:bool)
                n195 = case shown="True" w309 {
                  tunnel: [w311 "Ready"] -> w306
                  tunnel: w308 -> [w312 _]
                  tunnel: w307 -> [w317 _]
                  frame False {
                    n196 = Number To Decimal String(number=w317) -> (decimal integer string=w316:string)  [unwired: 1 in]
                    n197 = Concatenate Strings(w316, ", ") -> (w313:string)
                    n198 = Concatenate Strings(w313, w312) -> (w314:string)
                    n199 = Concatenate Strings("Error Setting Cleans: Code= ", w314) -> (w311:string)
                  }
                  frame True {
                    n200 = property on="Write INI Flag" class="Bool (strict)"("Value"=TRUE) -> ()  [unwired: 2 in, 2 out]
                  }
                }
                n201 = property on="Write Status" class="Str"("Value"=w306) -> ()  [unwired: 2 in, 2 out]
              }
            }
          }
        }
        n202 = case shown="True" w124 {
          tunnel: w125 -> [w224 w228]
          tunnel: [w224 w225] -> w122
          frame False {
          }
          frame True {
            n203 = flat-sequence {
              tunnel: w228 -> [w230]
              tunnel: [w230] -> w227
              tunnel: w227 -> [w245]
              tunnel: [w250] -> w226
              tunnel: w226 -> [w268]
              tunnel: [w268] -> w225
              frame #0 {
                n204 = property on="Write Status" class="Str"("Value"="Setting Custom Chip Values") -> ()  [unwired: 2 in, 2 out]
              }
              frame #1 {
                n205 = property on="Pre Y" class="DigNum (strict)"() -> ("Value"=w236:u32)  [unwired: 2 in, 2 out]
                n206 = property on="Post Y" class="DigNum (strict)"() -> ("Value"=w235:u32)  [unwired: 2 in, 2 out]
                n207 = property on="Active Y Size" class="DigNum (strict)"() -> ("Value"=w234:u32)  [unwired: 2 in, 2 out]
                n208 = property on="Pre X" class="DigNum (strict)"() -> ("Value"=w232:u32)  [unwired: 2 in, 2 out]
                n209 = property on="Post X" class="DigNum (strict)"() -> ("Value"=w231:u32)  [unwired: 2 in, 2 out]
                n210 = property on="Active X Size" class="DigNum (strict)"() -> ("Value"=w233:u32)  [unwired: 2 in, 2 out]
                n211 = Bundle By Name(cluster=T3 {"Pre Y"=0, "Post Y"=0, "Parallel (Y) Size"=0, "Pre X"=0, "Post X"=0, "Serial (X) Size"=0} ("Custom Chip Settings"), "Pre Y"=w236, "Post Y"=w235, "Parallel (Y) Size"=w234, "Pre X"=w232, "Post X"=w231, "Serial (X) Size"=w233) -> (w239:T3)
                n212 = property on="Enable / Disable Custom Chip" class="Bool (strict)"() -> ("Value"=w238:bool)  [unwired: 2 in, 2 out]
                n213 = property on="ReadOut Mode" class="Ring (strict)"() -> ("Value"=w248:u16)  [unwired: 2 in, 2 out]
                n214 = property on="Kinetics Window Height" class="DigNum (strict)"() -> ("Value"=w244:u32)  [unwired: 2 in, 2 out]
                n215 = property on="Timing Mode" class="Ring (strict)"() -> ("Value"=w243:u32)  [unwired: 2 in, 2 out]
                n216 = Equal?(x=w248, y=10) -> (x = y?=w247:bool)
                n217 = global read "CamHandle.vi" "Cam Handle"() -> (w242:u32)
                n218 = case shown="False" w247 {
                  tunnel: w245 -> [w256 w263]
                  tunnel: [w255 w262] -> w241
                  tunnel: w244 -> [_ w260]
                  tunnel: w243 -> [_ w259]
                  tunnel: w242 -> [w254 w258]
                  tunnel: w239 -> [w253 _]
                  tunnel: w238 -> [w252 _]
                  tunnel: [w251 w257] -> w237
                  frame False {
                    n219 = call <userlib>:"CameraSetCustomChip.vi"("error in (no error)"=w256, "Custom Chip Settings"=w253, "Enable/Disable Custom Chip"=w252, "Camera Handle"=w254) -> ("error out"=w255:errorcluster, "Camera Handle"=w251:u32)
                  }
                  frame True {
                    n220 = call <userlib>:"CameraKinetics.vi"("Camera Handle"=w258, "Window Size"=w260, "TriggerMode"=w259, "error in (no error)"=w263, "Enable/Disable Kinetics"=TRUE) -> ("Camera Handle"=w257:u32, "error out"=w262:errorcluster)
                  }
                }
                n221 = property on="Vertical Timing Index" class="DigNum (strict)"() -> ("Value"=w249:u32)  [unwired: 2 in, 2 out]
                n222 = call <userlib>:"CameraSetVertClk.vi"("error in (no error)"=w241, "Vertical Clock"=w249, "Camera Handle"=w237) -> ("error out"=w250:errorcluster)  [unwired: 1 out]
              }
              frame #2 {
                n223 = Unbundle By Name(w268) -> ("code"=w265:i32, "source"=w266:string)
                n224 = Equal To 0?(x=w265) -> (x = 0?=w267:bool)
                n225 = case shown="False" w267 {
                  tunnel: [w269 "Ready"] -> w264
                  tunnel: w266 -> [w270 _]
                  tunnel: w265 -> [w275 _]
                  frame False {
                    n226 = Number To Decimal String(number=w275) -> (decimal integer string=w274:string)  [unwired: 1 in]
                    n227 = Concatenate Strings(w274, ", ") -> (w271:string)
                    n228 = Concatenate Strings(w271, w270) -> (w272:string)
                    n229 = Concatenate Strings("Error Setting Clustom Chip: Code= ", w272) -> (w269:string)
                  }
                  frame True {
                    n230 = property on="Write INI Flag" class="Bool (strict)"("Value"=TRUE) -> ()  [unwired: 2 in, 2 out]
                  }
                }
                n231 = property on="Write Status" class="Str"("Value"=w264) -> ()  [unwired: 2 in, 2 out]
              }
            }
          }
        }
        n232 = Or(x="Set camera", y="Apply Logic Out") -> (x .or. y?=w121:bool)
        n233 = case shown="True" w121 {
          tunnel: w122 -> [w193 w197]
          tunnel: [w193 w194] -> w115
          frame False {
          }
          frame True {
            n234 = flat-sequence {
              tunnel: w197 -> [w199]
              tunnel: [w199] -> w196
              tunnel: w196 -> [w204]
              tunnel: [w200] -> w195
              tunnel: w195 -> [w213]
              tunnel: [w213] -> w194
              frame #0 {
                n235 = property on="Write Status" class="Str"("Value"="Setting Logic Out") -> ()  [unwired: 2 in, 2 out]
              }
              frame #1 {
                # "Filter Out\n\"Not Supported\"\n Warnings"
                n236 = property on="Invert" class="Bool (strict)"() -> ("Value"=w206:bool)  [unwired: 2 in, 2 out]
                n237 = global read "CamHandle.vi" "Cam Handle"() -> (w203:u32)
                n238 = property on="Logic Output" class="Ring (strict)"() -> ("Value"=w208:u16)  [unwired: 2 in, 2 out]
                n239 = Boolean To (0,1)(Boolean=w206) -> (0, 1=w207:i16)
                n240 = call <userlib>:"CameraSetLogic.vi"("Reserved"=0.0, "error in (no error)"=w204, "Invert Logic"=w207, "Logic Output"=w208, "Camera Handle"=w203) -> ("error out"=w201:errorcluster)  [unwired: 1 in, 1 out]
                n241 = call "FilterErrors.vi"("error in (no error)"=w201, "Error Numbers To Filter"="5007,5008") -> ("error out"=w200:errorcluster)
              }
              frame #2 {
                n242 = Unbundle By Name(w213) -> ("code"=w210:i32, "source"=w211:string)
                n243 = Equal To 0?(x=w210) -> (x = 0?=w212:bool)
                n244 = case shown="True" w212 {
                  tunnel: [w214 "Ready"] -> w209
                  tunnel: w211 -> [w215 _]
                  tunnel: w210 -> [w220 _]
                  frame False {
                    n245 = Number To Decimal String(number=w220) -> (decimal integer string=w219:string)  [unwired: 1 in]
                    n246 = Concatenate Strings(w219, ", ") -> (w216:string)
                    n247 = Concatenate Strings(w216, w215) -> (w217:string)
                    n248 = Concatenate Strings("Error Setting Logic Out Code= ", w217) -> (w214:string)
                  }
                  frame True {
                    n249 = property on="Write INI Flag" class="Bool (strict)"("Value"=TRUE) -> ()  [unwired: 2 in, 2 out]
                  }
                }
                n250 = property on="Write Status" class="Str"("Value"=w209) -> ()  [unwired: 2 in, 2 out]
              }
            }
          }
        }
        n251 = Or(x="Set camera", y="Apply ROI") -> (x .or. y?=w109:bool)
        n252 = property on="Enable / Disable Custom Chip" class="Bool (strict)"() -> ("Value"=w118:bool)  [unwired: 2 in, 2 out]
        n253 = case shown="False" w118 {
          tunnel: [w151 w167] -> w117
          tunnel: [w150 w166] -> w116
          tunnel: w115 -> [w149 w165]
          tunnel: [w147 w163] -> w114
          frame False {
            n254 = global read "CamHandle.vi" "X dimension"() -> (w152:u32)
            n255 = property on="ReadOut Mode" class="Ring (strict)"(error in=w149) -> (error out=w148:errorcluster, "Value"=w153:u16)  [unwired: 1 in, 1 out]
            n256 = Equal?(x=w153, y=10) -> (x = y?=w154:bool)
            n257 = case shown="True" w154 {
              tunnel: w152 -> [w158 w162]
              tunnel: [w158 w162] -> w151
              tunnel: [w157 w161] -> w150
              tunnel: w148 -> [w156 w160]
              tunnel: [w156 w159] -> w147
              frame False {
                n258 = global read "CamHandle.vi" "Y dimension"() -> (w157:u32)
              }
              frame True {
                n259 = property on="Kinetics Window Height" class="DigNum (strict)"(error in=w160) -> (error out=w159:errorcluster, "Value"=w161:u32)  [unwired: 1 in, 1 out]
              }
            }
          }
          frame True {
            n260 = property on="Active X Size" class="DigNum (strict)"(error in=w165) -> (error out=w164:errorcluster, "Value"=w167:u32)  [unwired: 1 in, 1 out]
            n261 = property on="Active Y Size" class="DigNum (strict)"(error in=w164) -> (error out=w163:errorcluster, "Value"=w166:u32)  [unwired: 1 in, 1 out]
          }
        }
        n262 = case shown="True" w109 {
          tunnel: [w168 w169] -> w113
          tunnel: w114 -> [w168 w182]
          frame False {
          }
          frame True {
            n263 = property on="X Start" class="DigNum (strict)"() -> ("Value"=w178:u32)  [unwired: 2 in, 2 out]
            n264 = property on="X End" class="DigNum (strict)"() -> ("Value"=w177:u32)  [unwired: 2 in, 2 out]
            n265 = property on="X Bin" class="DigNum (strict)"() -> ("Value"=w176:u32)  [unwired: 2 in, 2 out]
            n266 = property on="Y Start" class="DigNum (strict)"() -> ("Value"=w175:u32)  [unwired: 2 in, 2 out]
            n267 = property on="Y End" class="DigNum (strict)"() -> ("Value"=w174:u32)  [unwired: 2 in, 2 out]
            n268 = property on="Y Bin" class="DigNum (strict)"() -> ("Value"=w173:u32)  [unwired: 2 in, 2 out]
            n269 = Bundle("Value"=w178, "Value"=w177, "Value"=w176, "Value"=w175, "Value"=w174, "Value"=w173) -> (w181:T11)  [unwired: 1 in]
            n270 = global read "CamHandle.vi" "Cam Handle"() -> (w180:u32)
            n271 = call <userlib>:"CameraROI.vi"("error in"=w182, "ROI Params"=w181, "ROI Index"=1, "Camera Handle"=w180) -> ("error out"=w169:errorcluster)  [unwired: 1 out]
            n272 = Unbundle By Name(w169) -> ("code"=w171:i32, "source"=w170:string)
            n273 = Equal To 0?(x=w171) -> (x = 0?=w172:bool)
            n274 = case shown="False" w172 {
              tunnel: [w183 "Ready"] -> _
              tunnel: w170 -> [w184 _]
              tunnel: w171 -> [w189 _]
              frame False {
                n275 = Number To Decimal String(number=w189) -> (decimal integer string=w188:string)  [unwired: 1 in]
                n276 = Concatenate Strings(w188, ", ") -> (w185:string)
                n277 = Concatenate Strings(w185, w184) -> (w186:string)
                n278 = Concatenate Strings("Error Setting ROI. Code = ", w186) -> (w183:string)
              }
              frame True {
                n279 = property on="Write INI Flag" class="Bool (strict)"("Value"=TRUE) -> ()  [unwired: 2 in, 2 out]
              }
            }
          }
        }
        n280 = property on="X Size ROI" class="DigNum (strict)"("Value"=w117) -> ()  [unwired: 2 in, 2 out]
        n281 = property on="Y Size ROI" class="DigNum (strict)"("Value"=w116) -> ()  [unwired: 2 in, 2 out]
        n282 = property on="Write INI Flag" class="Bool (strict)"() -> ("Value"=w119:bool)  [unwired: 2 in, 2 out]
        n283 = case shown="True" w119 {
          tunnel: w113 -> [w381 w408]
          tunnel: [w381 w406] -> w142
          frame False {
            n284 = Wait Until Next ms Multiple(millisecond multiple=u32 10) -> ()  [unwired: 1 out]
          }
          frame True {
            n285 = global read "CamHandle.vi" "Cam Handle"() -> (w394:u32)
            n286 = call <userlib>:"CameraInitialize.vi"("error in"=w408, "Camera Handle"=w394) -> ("error out"=w409:errorcluster)  [unwired: 1 out]
            n287 = property on="Shutter State" class="Ring (strict)"() -> ("Value"=w430:u16)  [unwired: 2 in, 2 out]
            n288 = property on="Open" class="DigNum (strict)"() -> ("Value"=w431:u32)  [unwired: 2 in, 2 out]
            n289 = property on="Close" class="DigNum (strict)"() -> ("Value"=w432:u32)  [unwired: 2 in, 2 out]
            n290 = property on="Logic Output" class="Ring (strict)"() -> ("Value"=w433:u16)  [unwired: 2 in, 2 out]
            n291 = property on="Invert" class="Bool (strict)"() -> ("Value"=w434:bool)  [unwired: 2 in, 2 out]
            n292 = property on="Pre Y" class="DigNum (strict)"() -> ("Value"=w403:u32)  [unwired: 2 in, 2 out]
            n293 = property on="Post Y" class="DigNum (strict)"() -> ("Value"=w395:u32)  [unwired: 2 in, 2 out]
            n294 = property on="Active Y Size" class="DigNum (strict)"() -> ("Value"=w398:u32)  [unwired: 2 in, 2 out]
            n295 = property on="Pre X" class="DigNum (strict)"() -> ("Value"=w402:u32)  [unwired: 2 in, 2 out]
            n296 = property on="Post X" class="DigNum (strict)"() -> ("Value"=w396:u32)  [unwired: 2 in, 2 out]
            n297 = property on="Active X Size" class="DigNum (strict)"() -> ("Value"=w401:u32)  [unwired: 2 in, 2 out]
            n298 = property on="Enable / Disable Custom Chip" class="Bool (strict)"() -> ("Value"=w400:bool)  [unwired: 2 in, 2 out]
            n299 = property on="Vertical Timing Index" class="DigNum (strict)"() -> ("Value"=w399:u32)  [unwired: 2 in, 2 out]
            n300 = Bundle By Name(cluster=T8 {"Shutter State"=2, "Open Comp Time "=0, "Close Comp Time"=0, "Logic Out Setting"=1, "Logic Out Invert"=FALSE} ("Shutter and Logic Out"), "Shutter State"=w430, "Open Comp Time"=w431, "Close Comp Time"=w432, "Logic Out Setting"=w433, "Logic Out Invert"=w434) -> (w435:T8)
            n301 = property on="Speed" class="DigNum (strict)"() -> ("Value"=w427:i32)  [unwired: 2 in, 2 out]
            n302 = property on="Gain" class="Ring (strict)"() -> ("Value"=w426:i32)  [unwired: 2 in, 2 out]
            n303 = property on="Offset" class="DigNum (strict)"() -> ("Value"=w424:i32)  [unwired: 2 in, 2 out]
            n304 = property on="Readout Port" class="Ring (strict)"() -> ("Value"=w422:i32)  [unwired: 2 in, 2 out]
            n305 = property on="Number of Clean/Clears cycles" class="DigNum (strict)"() -> ("Value"=w421:u32)  [unwired: 2 in, 2 out]
            n306 = property on="Clean cycle height (Number of \nStrips per Clean/Clear)" class="DigNum (strict)"() -> ("Value"=w420:u32)  [unwired: 2 in, 2 out]
            n307 = property on="Final Section Height\n(Minimum Block Size)" class="DigNum (strict)"() -> ("Value"=w418:u32)  [unwired: 2 in, 2 out]
            n308 = property on="Final Section Count\n(Number of Minimum Blocks)" class="DigNum (strict)"() -> ("Value"=w419:u32)  [unwired: 2 in, 2 out]
            n309 = property on="Continous Cleans" class="Bool (strict)"() -> ("Value"=w423:bool)  [unwired: 2 in, 2 out]
            n310 = property on="Skip Serial Register Clean" class="Bool (strict)"() -> ("Value"=w425:bool)  [unwired: 2 in, 2 out]
            n311 = Bundle By Name(cluster=T5 {"Pre Y"=0, "Post Y"=0, "Active Y"=0, "Pre X"=0, "Post X"=0, "Active X"=0, "Custom Chip Enabled"=FALSE, "Vertical Timing Index"=0} ("Custom Chip"), "Pre Y"=w403, "Post Y"=w395, "Active Y"=w398, "Pre X"=w402, "Post X"=w396, "Active X"=w401, "Custom Chip Enabled"=w400, "Vertical Timing Index"=w399) -> (w397:T5)
            n312 = Bundle By Name(cluster=T7 {"ADC Speed"=-2, "ADC Gain"=-1, "ADC Offset"=-1, "Readout Port"=-1, "Num Cleans"=1, "Num Strips per Clean"=10, "Mini Block Size"=2, "Num Min Blocks"=3, "Continous Cleans"=FALSE, "Skip Serial Reg Clean"=FALSE} ("ADC and Cleans"), "ADC Speed"=w427, "ADC Gain"=w426, "ADC Offset"=w424, "Readout Port"=w422, "Num Cleans"=w421, "Num Strips per Clean"=w420, "Mini Block Size"=w418, "Num Min Blocks"=w419, "Continous Cleans"=w423, "Skip Serial Reg Clean"=w425) -> (w428:T7)
            n313 = property on="Camera Number" class="DigNum (strict)"() -> ("Value"=w410:u32)  [unwired: 2 in, 2 out]
            n314 = property on="Camera Number" class="DigNum (strict)"() -> ("Value"=w391:u32)  [unwired: 2 in, 2 out]
            n315 = property on="X Start" class="DigNum (strict)"() -> ("Value"=w389:u32)  [unwired: 2 in, 2 out]
            n316 = property on="X End" class="DigNum (strict)"() -> ("Value"=w388:u32)  [unwired: 2 in, 2 out]
            n317 = property on="X Bin" class="DigNum (strict)"() -> ("Value"=w387:u32)  [unwired: 2 in, 2 out]
            n318 = property on="Y Start" class="DigNum (strict)"() -> ("Value"=w386:u32)  [unwired: 2 in, 2 out]
            n319 = property on="Y End" class="DigNum (strict)"() -> ("Value"=w385:u32)  [unwired: 2 in, 2 out]
            n320 = property on="Y Bin" class="DigNum (strict)"() -> ("Value"=w384:u32)  [unwired: 2 in, 2 out]
            n321 = property on="Exposure" class="DigNum (strict)"() -> ("Value"=w411:dbl)  [unwired: 2 in, 2 out]
            n322 = property on="Collection Mode" class="Ring (strict)"() -> ("Value"=w412:u32)  [unwired: 2 in, 2 out]
            n323 = property on="Timing Mode" class="Ring (strict)"() -> ("Value"=w413:u32)  [unwired: 2 in, 2 out]
            n324 = property on="Trigger Edge" class="Ring (strict)"() -> ("Value"=w414:u32)  [unwired: 2 in, 2 out]
            n325 = property on="Temperature" class="DigNum (strict)"() -> ("Value"=w415:dbl)  [unwired: 2 in, 2 out]
            n326 = Bundle By Name(cluster=T4 {"Camera Number"=0, "ROI Number"=0, "X Start"=0, "X End"=0, "X Bin"=0, "Y Start"=0, "Y End"=0, "Y Bin"=0} ("ROI Values"), "Camera Number"=w391, "ROI Number"=1, "X Start"=w389, "X End"=w388, "X Bin"=w387, "Y Start"=w386, "Y End"=w385, "Y Bin"=w384) -> (w383:T4)
            n327 = Bundle By Name(cluster=T6 {"Exposure"=0.001, "Collection Mode"=1, "Timing Mode"=1, "Trigger Edge"=1, "Temperature"=-10.0} ("Timing and Temperature"), "Exposure"=w411, "Collection Mode"=w412, "Timing Mode"=w413, "Trigger Edge"=w414, "Temperature"=w415) -> (w416:T6)
            n328 = call "WriteCameraSetupToIni.vi"("ADC and Cleans"=w428, "Camera Number"=w410, "Shutter and Logic Out"=w435, "Custom Chip"=w397, "error in (no error)"=w409, "Timing and Temperature"=w416) -> ("error out"=w407:errorcluster)  [unwired: 2 in]
            n329 = call "WriteOneHwROIToIni.vi"("error in (no error)"=w407, "Show Message"=FALSE, "ROI Values"=w383) -> ("error out"=w393:errorcluster)
            n330 = property on="Write INI Flag" class="Bool (strict)"(error in=w393, "Value"=FALSE) -> (error out=w406:errorcluster)  [unwired: 1 in, 1 out]
          }
        }
        n331 = case shown="True" "Read Camera settings" {
          tunnel: w142 -> [w509 w518]
          tunnel: [w509 w515] -> w141
          frame False {
          }
          frame True {
            w539 = 30  # SICAMERA_READOUT_TIME
            n332 = property on="Exposure" class="DigNum (strict)"() -> ("Value"=w517:dbl)  [unwired: 2 in, 2 out]
            n333 = property on="Frames to collect (nframe)" class="DigNum (strict)"() -> ("Value"=w513:u32)  [unwired: 2 in, 2 out]
            n334 = global read "CamHandle.vi" "Cam Handle"() -> (w519:u32)
            n335 = property on="Collection Mode" class="Ring (strict)"() -> ("Value"=w511:u32)  [unwired: 2 in, 2 out]
            n336 = call <userlib>:"CameraExperiment.vi"("Number of Accumulations"=1, "Acquire / Focus Flag"=w511, "error in"=w518, "Number of Images"=w513, "Exposure (sec)"=w517, "Camera Handle"=w519) -> ("error out"=w521:errorcluster, "Camera Handle"=w520:u32)
            n337 = call <userlib>:"CameraInitialize.vi"("error in"=w521, "Camera Handle"=w520) -> ("error out"=w523:errorcluster, "Camera Handle"=w522:u32)
            n338 = call <userlib>:"CameraADCget.vi"("Camera handle"=w522, "error in (no error)"=w523) -> ("Bit Depth"=→"Bit Depth":i32, "Pixel Time"=→"Pixel Time\n(1/ADC Speed)":i32, "Readout Port"=→"ReadOut Port":i32, "ADC Offset"=→"ADC Offset":i32, "Camera handle"=w540:u32, "ADC Speed"=→"ADC Speed":i32, "ADC Gain"=→"ADC Gain":i32, "error out"=w541:errorcluster)
            n339 = call <userlib>:"CameraGetTemp.vi"("Camera Handle"=w540, "error in (no error)"=w541) -> ("Camera Handle"=w537:u32, "Temperature"=→"Temperature 2" →"Thermometer":dbl, "error out"=w538:errorcluster)
            n340 = call <userlib>:"CameraGetVar.vi"("error in"=w538, "Parameter ID"=w539, "Camera Handle"=w537) -> ("error out"=w529:errorcluster, "Value"=→"Readout Time":dbl, "Camera Handle"=w527:u32)
            n341 = call <userlib>:"CameraGetVar.vi"("error in"=w529, "Parameter ID"=252, "Camera Handle"=w527) -> ("error out"=w528:errorcluster, "Value"=→"Frame Rate Calc":dbl, "Camera Handle"=w526:u32)
            n342 = call <userlib>:"CameraGetCustomChip.vi"("Camera Handle"=w526, "error in (no error)"=w528) -> ("Camera Handle"=w533:u32, "Custum chip Enable/Disable status"=→"Custom Chip Enabled":bool, "error out"=w532:errorcluster)  [unwired: 1 out]
            n343 = call <userlib>:"CameraGetVertClkInfo.vi"("Camera Handle"=w533, "error in (no error)"=w532) -> ("VertClk index"=→"Vertical Index":u32, "Real Clock Value"=→"Vertical Timing":dbl, "error out"=w516:errorcluster)  [unwired: 3 out]
            n344 = call "FilterErrors.vi"("error in (no error)"=w516, "Error Numbers To Filter"="5011") -> ("error out"=w515:errorcluster)
          }
        }
      }
      "error out" <- w23
    }
    frame #1 {
      n345 = stacked-sequence {
        seq-local: [w547 _ _] -> [_ w549 _]
        seq-local: [w548 _ _] -> [_ w552 _]
        seq-local: [_ w551 _] -> [_ _ w914]
        seq-local: [_ w550 _] -> [_ _ w913]
        frame #0 {
          n346 = global read "CamHandle.vi" "Cam Handle"() -> (w548:u32)
          n347 = local read "error out"() -> (w547:errorcluster)
        }
        frame #1 {
          n348 = while {
            tunnel: w552 -> [w562]
            tunnel: w549 -> [w554]
            tunnel: [w558] -> w551
            tunnel: [w557] -> w550
            stop <- w555 stop-if-true
            n349 = stacked-sequence {
              seq-local: [_ w665 _] -> [_ _ w750]
              seq-local: [_ w664 _] -> [_ _ w752]
              seq-local: [w567 _ _] -> [_ w662 _]
              seq-local: [w568 _ _] -> [_ w663 _]
              tunnel: w562 -> [w565 _ _]
              tunnel: w554 -> [w572 _ _]
              tunnel: "?" -> [w569 w670 w756]
              tunnel: "Number of Images" -> [_ w668 w753]
              tunnel: "Timepoints" -> [_ _ w745]
              tunnel: [_ _ w749] -> w558
              tunnel: [_ _ w748] -> w557
              tunnel: "# of Sets" -> [_ _ w746]
              frame #0 {
                n350 = Equal?(x=w569, y=T9."RUN") -> (x = y?=w566:bool)
                n351 = case shown="False" "?" {
                  tunnel: w572 -> [w578 w610]
                  tunnel: [w575 w613] -> w567
                  tunnel: [w577 w612] -> w568
                  tunnel: w566 -> [_ _]
                  tunnel: w565 -> [w576 w611]
                  tunnel: "Exposure Time (s)" -> [w574 w608]
                  frame False {
                    n352 = case shown="False" "?" {
                      tunnel: w578 -> [w580 w592]
                      tunnel: [w580 w591] -> w577
                      tunnel: w576 -> [w579 w593]
                      tunnel: [w579 w590] -> w575
                      tunnel: w574 -> [_ w594]
                      frame False {
                      }
                      frame True {
                        n353 = Path To String(path="file path") -> (string=w586:string)
                        n354 = Concatenate Strings(w586, "\\" ("string"), "File_name", "_" ("string")) -> (w581:string)
                        n355 = for {
                          N: "# of Frames" -> [_]
                          tunnel: w594 -> [w607]
                          tunnel: w593 -> [w606]
                          tunnel: w592 -> [w605]
                          tunnel: [w604] -> w591
                          tunnel: [w603] -> w590
                          tunnel: "# of spectrum per frame" -> [w602]
                          tunnel: w581 -> [w598]
                          i -> [w595]
                          n356 = Number To Decimal String(number=w595) -> (decimal integer string=w597:string)  [unwired: 1 in]
                          n357 = call "avarage_images.vi"("error in (no error)"=w605, "Exposure Time (s)"=w607, "Number of Images"=w602, "Camera Handle"=w606) -> ("error out"=w604:errorcluster, "Camera Handle"=w603:u32, "Waveform Graph"=w601:i32[])  [unwired: 3 in, 2 out]
                          n358 = Concatenate Strings(w598, w597) -> (w596:string)
                          n359 = String To Path(string=w596) -> (path=w599:path)
                          n360 = local write item#17(w601) -> ()
                          n361 = call-poly <vilib>:"Write To Spreadsheet File.vi"("transpose? (no:F)"=TRUE, "1D data"=w601, "file path (dialog if empty)"=w599) -> ()  [unwired: 5 in, 1 out]
                        }
                        n362 = local write "PyLoN Ready"(FALSE ("PyLoN Ready")) -> ()
                      }
                    }
                  }
                  frame True {
                    w615 = u32 1  # acquire focus mode
                    w616 = u32 1  # Software accumulation
                    # "focus mode (1) ->"
                    # "This is similar to \"Run\"  in Lightfield\nTrigger mode= internal"
                    n363 = call "ExSubImageCreate.vi"("Camera Handle"=w611, "error in (no error)"=w610) -> ("Camera Handle"=w617:u32, "Data Handle"=w623:u32, "error out"=w618:errorcluster)
                    n364 = Bundle("acquire focus mode"=w615, "Exposure Time (s)"=w608, 1, "Software accumulation"=w616) -> (w614:T12)  [unwired: 1 in]
                    n365 = call "ExSubInitCam.vi"("error in (no error)"=w618, "Camera Information"=w614, "Camera Handle"=w617) -> ("error out"=w619:errorcluster, "Camera Handle"=w620:u32)
                    n366 = call <userlib>:"CameraStart.vi"("error in"=w619, "Camera Handle"=w620) -> ("error out"=w621:errorcluster, "Camera Handle"=w622:u32)
                    n367 = while {
                      tunnel: [w638] -> w624
                      tunnel: [w637] -> w626
                      tunnel: [w636] -> w625
                      tunnel: w621 -> [w635]
                      tunnel: w622 -> [w634]
                      tunnel: w623 -> [w633]
                      stop <- "?" stop-if-true
                      n368 = call <userlib>:"CameraCheckData.vi"("Camera Handle"=w634, "error in"=w635) -> ("Camera Handle"=w640:u32, "Number Of Frames Available"=w642:i32, "error out"=w639:errorcluster)
                      n369 = Greater Than 0?(x=w642) -> (x > 0?=w641:bool)
                      n370 = case shown="True" w641 {
                        selector: w641 -> [w645 w658]
                        tunnel: w640 -> [w643 w660]
                        tunnel: w639 -> [w646 w659]
                        tunnel: [w645 w658] -> _
                        tunnel: [w646 w657] -> w637
                        tunnel: w633 -> [w644 w651]
                        tunnel: [w644 w655] -> w638
                        tunnel: [w643 w654] -> w636
                        frame False {
                        }
                        frame True {
                          w656 = 1
                          n371 = call <userlib>:"CameraGetData.vi"("error in"=w659, "Image/Data Handle"=w651, "Camera Handle"=w660) -> ("error out"=w653:errorcluster, "Image/Data Handle"=w652:u32, "Camera Handle"=w654:u32)
                          n372 = call <userlib>:"ImageGetLineU16.vi"("Data Handle"=w652, "Y Position"=w656, "Z Position"=w656, "error in"=w653) -> ("Array u16"=w650:u16[], "Data Handle"=w655:u32, "error out"=w657:errorcluster)
                          n373 = Delete From Array(array=w650, length=2, index=0) -> (array with subset deleted=→"?":u16[])  [unwired: 1 out]
                        }
                      }
                    }
                    n374 = local write "PyLoN Ready"(FALSE ("PyLoN Ready")) -> ()
                    n375 = call <userlib>:"ImageDestroy.vi"("error in"=w626, "Data handle"=w624) -> ()  [unwired: 1 out]
                    n376 = stacked-sequence {
                      tunnel: w626 -> [w631]
                      tunnel: w625 -> [w630]
                      tunnel: [w629] -> w612
                      tunnel: [w628] -> w613
                      frame #0 {
                        n377 = call <userlib>:"CameraStop.vi"("error in"=w631, "Camera Handle"=w630) -> ("error out"=w629:errorcluster, "Camera Handle"=w628:u32)
                        n378 = call <vilib>:"Beep.vi"() -> ()  [unwired: 12 in]
                      }
                    }
                  }
                }
                "PyLoN Ready" <- TRUE
              }
              frame #1 {
                n379 = Equal?(x=w670, y=T2."FOCUS") -> (x = y?=w666:bool)
                n380 = And(x=w666, y="?") -> (x .and. y?=w669:bool)
                n381 = case shown="True" w669 {
                  tunnel: w662 -> [w678 w727]
                  tunnel: [w674 w726] -> w665
                  tunnel: w663 -> [w676 w725]
                  tunnel: w668 -> [w677 w724]
                  tunnel: [w675 w723] -> w664
                  tunnel: w666 -> [w671 _]
                  frame False {
                    n382 = And(x=w671, y="?") -> (x .and. y?=w673:bool)
                    n383 = case shown="False" w673 {
                      tunnel: w678 -> [w681 w707]
                      tunnel: w677 -> [w682 w706]
                      tunnel: w676 -> [w683 w705]
                      tunnel: [w679 w704] -> w675
                      tunnel: [w680 w703] -> w674
                      tunnel: w671 -> [w684 _]
                      frame False {
                        n384 = And(x=w684, y="?") -> (x .and. y?=w686:bool)
                        n385 = case shown="False" w686 {
                          tunnel: w683 -> [w687 w692]
                          tunnel: w682 -> [_ w695]
                          tunnel: w681 -> [w688 w694]
                          tunnel: [w688 w690] -> w680
                          tunnel: [w687 w691] -> w679
                          frame False {
                          }
                          frame True {
                            # "Acquire"
                            n386 = local read "FLIP SPECTRA"() -> (w697:bool)
                            n387 = Initialize Array(0.0, u32 1340) -> (w693:dbl[])
                            n388 = call "PyLoN_data.vi"("Number of Images"=w695, "error in (no error)"=w692, "PumpOffBkgd"=w693, "PumpOnBkgd"=w693, "Camera Handle"=w694) -> ("error out"=w691:errorcluster, "Camera Handle 2"=w690:u32, "Raman_Gain"=w689:dbl[])  [unwired: 1 in, 3 out]
                            n389 = case shown="False" w697 {
                              tunnel: w689 -> [w700 w702]
                              tunnel: [w700 w701] -> w696
                              frame False {
                              }
                              frame True {
                                n390 = Reciprocal(x=w702) -> (1/x=w701:dbl[])
                              }
                            }
                            n391 = local write item#11(w696) -> ()
                          }
                        }
                      }
                      frame True {
                        # "Winspec"
                        n392 = while {
                          tunnel: w707 -> [w713]
                          tunnel: w706 -> [w714]
                          tunnel: [w708] -> w703
                          tunnel: w705 -> [w712]
                          tunnel: [w711] -> w704
                          stop <- w717 stop-if-true
                          n393 = local read item#12() -> (w717:bool)
                          n394 = Initialize Array(0.0, u32 1340) -> (w709:dbl[])
                          n395 = local read "FLIP SPECTRA"() -> (w716:bool)
                          n396 = call "PyLoN_data.vi"("Number of Images"=w714, "error in (no error)"=w712, "PumpOffBkgd"=w709, "PumpOnBkgd"=w709, "Camera Handle"=w713) -> ("error out"=w711:errorcluster, "Pump_Off"=w710:dbl[], "Camera Handle 2"=w708:u32)  [unwired: 1 in, 3 out]
                          n397 = case shown="False" w716 {
                            tunnel: w710 -> [w720 w721]
                            tunnel: [w720 w722] -> w715
                            frame False {
                            }
                            frame True {
                              n398 = Reciprocal(x=w721) -> (1/x=w722:dbl[])
                            }
                          }
                          n399 = local write item#11(w715) -> ()
                        }
                      }
                    }
                  }
                  frame True {
                    # "Focus"
                    n400 = while {
                      tunnel: w725 -> [w733]
                      tunnel: w724 -> [w734]
                      tunnel: [w732] -> w723
                      tunnel: w727 -> [w735]
                      tunnel: [w730] -> w726
                      stop <- "?" stop-if-true
                      n401 = Initialize Array(0.0, u32 1021) -> (w731:dbl[])
                      n402 = call "PyLoN_data.vi"("Number of Images"=w734, "error in (no error)"=w733, "PumpOffBkgd"=w731, "PumpOnBkgd"=w731, "Camera Handle"=w735) -> ("error out"=w732:errorcluster, "Camera Handle 2"=w730:u32, "Raman_Gain"=w729:dbl[], "x/y"=→"x/y":dbl)  [unwired: 1 in, 2 out]
                      n403 = local read "FLIP SPECTRA"() -> (w737:bool)
                      n404 = case shown="False" w737 {
                        tunnel: w729 -> [w741 w743]
                        tunnel: [w741 w742] -> w736
                        frame False {
                        }
                        frame True {
                          n405 = Reciprocal(x=w743) -> (1/x=w742:dbl[])
                        }
                      }
                      "?" <- w736
                    }
                  }
                }
              }
              frame #2 {
                n406 = Array Size(array=w745) -> (size(s)=w744:i32)
                n407 = Equal?(x=w756, y=T2."FSRS") -> (x = y?=w754:bool)
                n408 = And(x="?", y=w754) -> (x .and. y?=w755:bool)
                n409 = case shown="True" w755 {
                  tunnel: w753 -> [_ w766]
                  tunnel: w750 -> [w757 w765]
                  tunnel: w752 -> [w758 w761]
                  tunnel: w745 -> [_ w764]
                  tunnel: [w757 w763] -> w749
                  tunnel: [w758 w762] -> w748
                  tunnel: w746 -> [_ w760]
                  tunnel: w744 -> [_ w759]
                  frame False {
                  }
                  frame True {
                    n410 = for {
                      N: w760 -> [_]
                      tunnel: w766 -> [w773]
                      tunnel: w765 -> [w772]
                      tunnel: w764 -> [w771]
                      tunnel: [w770] -> w763
                      tunnel: [w769] -> w762
                      tunnel: w761 -> [w768]
                      tunnel: w759 -> [w767]
                      n411 = stacked-sequence {
                        seq-local: [w776 _] -> [_ w786]
                        tunnel: w773 -> [_ w785]
                        tunnel: w772 -> [_ w784]
                        tunnel: [_ w780] -> _
                        tunnel: w771 -> [w774 w783]
                        tunnel: [_ w782] -> w769
                        tunnel: [_ w781] -> w770
                        tunnel: w768 -> [_ w780]
                        tunnel: w767 -> [_ w779]
                        frame #0 {
                          n412 = Array Size(array=w774) -> (size(s)=w778:i32)
                          n413 = call "randomize.vi"("Input array"=w774) -> ("Output array"=w775:dbl[])
                          n414 = Quotient & Remainder(x=w778, y="#Ground per set") -> (floor(x/y)=w776:u32)  [unwired: 1 out]
                          n415 = local write "Timepoints"(w775) -> ()
                        }
                        frame #1 {
                          n416 = for {
                            N: w779 -> [_]
                            tunnel: w786 -> [w793]
                            tunnel: w785 -> [w792]
                            tunnel: w784 -> [w791]
                            tunnel: w783 -> [w790]
                            tunnel: [w789] -> w782
                            tunnel: [w788] -> w781
                            tunnel: w780 -> [w787]
                            i -> [w794]
                            n417 = stacked-sequence {
                              seq-local: [w796 _] -> [_ w859]
                              seq-local: [w797 _] -> [_ w860]
                              seq-local: [w795 _] -> [_ w858]
                              tunnel: w794 -> [w798 w861]
                              tunnel: w793 -> [w803 _]
                              tunnel: w792 -> [w801 w863]
                              tunnel: w791 -> [w800 _]
                              tunnel: w787 -> [w799 _]
                              tunnel: w790 -> [_ w862]
                              tunnel: [_ w857] -> w789
                              tunnel: [_ w856] -> w788
                              frame #0 {
                                n418 = Quotient & Remainder(x=w798, y=w803) -> (x-y*floor(x/y)=w804:u32, floor(x/y)=w802:u32)
                                n419 = Equal To 0?(x=w804) -> (x = 0?=w805:bool)
                                n420 = case shown="True" w805 {
                                tunnel: w802 -> [_ w817]
                                tunnel: w801 -> [_ w821]
                                tunnel: w800 -> [w807 w820]
                                tunnel: w799 -> [w806 w819]
                                tunnel: [w807 w810] -> w796
                                tunnel: [w806 w809] -> w797
                                tunnel: w798 -> [_ w818]
                                tunnel: [_ w808] -> w795
                                frame False {
                                }
                                frame True {
                                n421 = flat-sequence {
                                tunnel: w821 -> [w842]
                                tunnel: w820 -> [w841]
                                tunnel: w819 -> [w840]
                                tunnel: w818 -> [w828]
                                tunnel: w817 -> [w826]
                                tunnel: [w839] -> w816
                                tunnel: [w838] -> w815
                                tunnel: [w835] -> w814
                                tunnel: [w834] -> w813
                                tunnel: [w823] -> w812
                                tunnel: [w822] -> w811
                                tunnel: w816 -> [w848]
                                tunnel: w815 -> [w847]
                                tunnel: w814 -> [w851]
                                tunnel: w813 -> [w850]
                                tunnel: w812 -> [w852]
                                tunnel: w811 -> [w846]
                                tunnel: [w848] -> w810
                                tunnel: [w847] -> w809
                                tunnel: [w846] -> w808
                                frame #0 {
                                w827 = "_" ("string")
                                n422 = local read "FLIP SPECTRA"() -> (w837:bool)
                                n423 = call "PyLoN_data.vi"("Number of Images"=w842, "error in (no error)"=w840, "Camera Handle"=w841) -> ("error out"=w838:errorcluster, "Pump_Off"=w834:dbl[], "Pump_On"=w835:dbl[], "Camera Handle 2"=w839:u32, "Raman_Gain"=w822:dbl[])  [unwired: 3 in, 1 out]
                                n424 = Format Into String(w828) -> (resulting string=w829:string)  [unwired: 3 in, 1 out]
                                n425 = Format Into String(w826) -> (resulting string=w825:string)  [unwired: 3 in, 1 out]
                                n426 = case shown="False" w837 {
                                tunnel: w822 -> [w843 w845]
                                tunnel: [w843 w844] -> w836
                                frame False {
                                }
                                frame True {
                                n427 = Reciprocal(x=w845) -> (1/x=w844:dbl[])
                                }
                                }
                                "?" <- w836
                                n428 = Path To String(path="File Path") -> (string=w833:string)
                                n429 = Concatenate Strings(w833, "\\" ("string"), "File Name", w827, w829, w827, w825, "gr" ("string")) -> (w823:string)
                                }
                                frame #1 {
                                n430 = String To Path(string=w852) -> (path=w853:path)
                                n431 = Build Array(w846, w851, w850) -> (w849:dbl[][])
                                n432 = call-poly <vilib>:"Write To Spreadsheet File.vi"("transpose? (no:F)"=TRUE, "format (%.3f)"="%.7f", "2D data"=w849, "file path (dialog if empty)"=w853) -> ()  [unwired: 4 in, 1 out]
                                }
                                }
                                }
                                }
                              }
                              frame #1 {
                                n433 = stacked-sequence {
                                seq-local: [_ w866 _ _ _] -> [_ _ _ w887 _]
                                seq-local: [_ w869 _ _ _] -> [_ _ _ w886 w893]
                                seq-local: [_ w868 _ _ _] -> [_ _ _ w885 _]
                                seq-local: [_ w867 _ _ _] -> [_ _ _ w884 _]
                                tunnel: w860 -> [_ w879 _ _ _]
                                tunnel: w859 -> [_ w878 _ _ _]
                                tunnel: w863 -> [_ w877 _ _ _]
                                tunnel: w862 -> [_ w874 _ _ _]
                                tunnel: w861 -> [_ w870 _ _ _]
                                tunnel: w858 -> [_ _ _ _ w894]
                                tunnel: [_ w865 _ _ _] -> w857
                                tunnel: [_ w864 _ _ _] -> w856
                                frame #0 {
                                }
                                frame #1 {
                                n434 = Index Array(array=w874, index=w870) -> (element=w873:dbl)
                                n435 = call "tppathcr.vi"("input"=w873) -> ("out"=w872:string)
                                n436 = local read "File Path"() -> (w876:path)
                                n437 = local read "File Name"() -> (w875:string)
                                n438 = call "PyLoN_data.vi"("Number of Images"=w877, "error in (no error)"=w879, "Camera Handle"=w878) -> ("error out"=w865:errorcluster, "Pump_Off"=w867:dbl[], "Pump_On"=w868:dbl[], "Camera Handle 2"=w864:u32, "Raman_Gain"=w869:dbl[])  [unwired: 3 in, 1 out]
                                n439 = Format Into String(w870) -> (resulting string=w880:string)  [unwired: 3 in, 1 out]
                                n440 = Path To String(path=w876) -> (string=w883:string)
                                n441 = Concatenate Strings(w883, "\\" ("string"), w875, "_" ("string"), w872, "exe" ("string"), w880) -> (w866:string)
                                }
                                frame #2 {
                                }
                                frame #3 {
                                n442 = String To Path(string=w887) -> (path=w889:path)
                                n443 = Build Array(w886, w885, w884) -> (w888:dbl[][])
                                n444 = call-poly <vilib>:"Write To Spreadsheet File.vi"("transpose? (no:F)"=TRUE, "format (%.3f)"="%.7f", "2D data"=w888, "file path (dialog if empty)"=w889) -> ()  [unwired: 4 in, 1 out]
                                }
                                frame #4 {
                                n445 = case shown="False" "Ground State\nSubstract?" {
                                tunnel: w894 -> [_ w903]
                                tunnel: w893 -> [w897 w902]
                                frame False {
                                n446 = local read "FLIP SPECTRA"() -> (w896:bool)
                                n447 = case shown="True" w896 {
                                tunnel: [w898 w900] -> w895
                                tunnel: w897 -> [w898 w899]
                                frame False {
                                }
                                frame True {
                                n448 = Reciprocal(x=w899) -> (1/x=w900:dbl[])
                                }
                                }
                                n449 = local write item#1(w895) -> ()
                                }
                                frame True {
                                n450 = local read "FLIP SPECTRA"() -> (w904:bool)
                                n451 = case shown="False" w904 {
                                tunnel: [w907 w912] -> w906
                                tunnel: w903 -> [w908 w909]
                                tunnel: [w908 w911] -> w905
                                tunnel: w902 -> [w907 w910]
                                frame False {
                                }
                                frame True {
                                n452 = Reciprocal(x=w910) -> (1/x=w912:dbl[])
                                n453 = Reciprocal(x=w909) -> (1/x=w911:dbl[])
                                }
                                }
                                n454 = Subtract(x=w906, y=w905) -> (x-y=w901:dbl[])
                                n455 = local write item#1(w901) -> ()
                                }
                                }
                                }
                                }
                              }
                            }
                          }
                        }
                      }
                    }
                  }
                }
              }
            }
            n456 = Or(x=w554, y="?") -> (x .or. y?=w555:bool)
          }
        }
        frame #2 {
          n457 = local write "PyLoN Ready"(FALSE ("PyLoN Ready")) -> ()
          n458 = call "ExSubCloseCamUnInit.vi"("error in (no error)"=w913, "Camera Handle"=w914) -> ("error out"=→"PyLoN Error Out":errorcluster)
        }
      }
    }
  }
